vi "SR430_set_discriminator_level.vi"(0 "address":T1, 2 "discriminatorLevel [V]":dbl format="%.2f", 5 "error in (no error)":errorcluster) -> (14 "address out":T1, 19 "error out":errorcluster)   [LabVIEW 2015, in "SR430Driver.lvlib"]
doc: "Sets the discriminator threshold level. That level must be within -0.3V <= x <=0.3V.\n\nCopyright (C)\nGesellschaft für Schwerionenforschung, GSI\nPlanckstr. 1\n64291 Darmstadt\nGermany\n\nContact: D.Beck@gsi.de \n\nThis program is free software; you can redistribute it and/or modify it under the terms of the \nGNU General Public License as published by the Free Software Foundation; either version 2 of the license, or (at your option) any later version.\n\nThis program is distributed in the hope that it will be useful, but WITHOUT ANY WARRANTY; without even the implied warranty of MERCHANTABILITY or FITNESS FOR A PARTICULAR PURPOSE. See the GNU General License for more details (http://www.gnu.org).\n\nGesellschaft für Schwerionenforschung, GSI\nPlanckstr. 1, 64291 Darmstadt, Germany\nFor all questions and ideas contact: M.Richter@gsi.de, K.Poppensieker, H.Brand@gsi.de or D.Beck@gsi.de.\nLast update: 11-APR-2002"
uses:
  SR430Driver.lvlib
  SR430_VISA Control.ctl
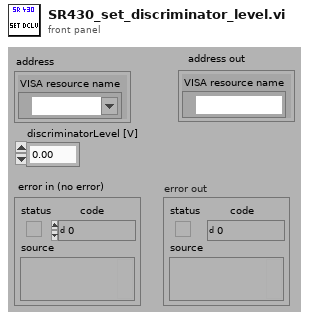
[diagram p1: front panel]
types:
  T1 = typedef "SR430Driver.lvlib/SR430_VISA Control.ctl" = cluster{"VISA resource name":refnum<visa-resource-name>}
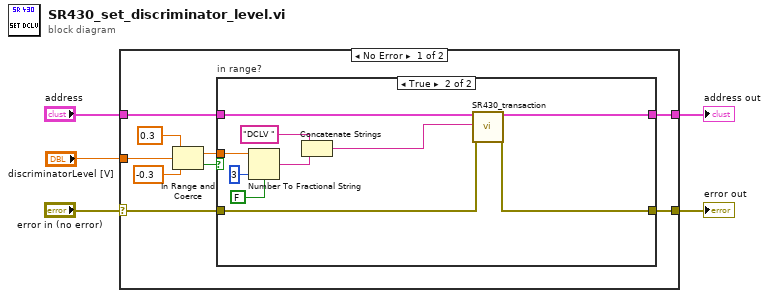
[diagram p0: block diagram]
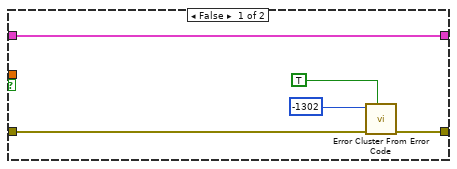
[diagram p2: hidden frame]
diagram:
  n1 = case shown="No Error" "error in (no error)" {
    selector: "error in (no error)" -> [w6 w30]
    tunnel: "address" -> [w14 w31]
    tunnel: [w13 w31] -> w4
    tunnel: [w12 w30] -> w3
    tunnel: "discriminatorLevel [V]" -> [w11 _]
    frame No Error {
      n2 = In Range and Coerce(upper limit=0.3, x=w11, lower limit=-0.3) -> (coerced(x)=w7:dbl, In Range?=w8:bool)
      n3 = case "in range?" shown="True" w8 {
        tunnel: w14 -> [w19 w25]
        tunnel: [w19 w23] -> w13
        tunnel: w6 -> [w17 w24]
        tunnel: [w18 w22] -> w12
        tunnel: w7 -> [_ w29]
        frame False {
          n4 = call <vilib>:"Error Cluster From Error Code.vi"("show call chain? (False)"=TRUE, "error in (no error)"=w17, "error code (0)"=-1302 ("code")) -> ("error out"=w18:errorcluster)  [unwired: 6 in]
        }
        frame True {
          n5 = Number To Fractional String(use system decimal point (T)=FALSE, number=w29, precision (6)=i16 3) -> (F-format string=w27:string)  [unwired: 1 in]
          n6 = Concatenate Strings("DCLV ", w27) -> (w21:string)
          n7 = call "SR430_transaction.vi"("SR430 VISA Cluster"=w25, "SR430 Command String"=w21, "error in (no error)"=w24) -> ("dup SR430 VISA Cluster"=w23:T1, "error out"=w22:errorcluster)  [unwired: 13 in, 2 out]
        }
      }
    }
    frame Error {
    }
  }
  "address out" <- w4
  "error out" <- w3
